vi "呈现图片.vi"(8 "error in (no error)":errorcluster caption="错误输入（无错误）", 11 "直线 输入":refnum<class "直线.lvclass"> caption="DNL_LabVIEW Object in") -> (0 "error out":errorcluster caption="错误输出", 2 "Picture":picture caption="图片", 3 "直线 输出":refnum<class "直线.lvclass"> caption="DNL_LabVIEW Object out")   [LabVIEW 2011, in "直线.lvclass"]
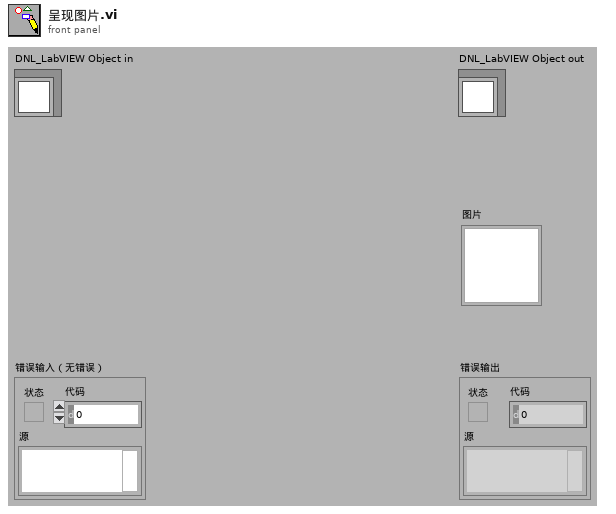
[diagram p1: front panel]
types:
  T1 = typedef "LVPointDoubleTypeDef.ctl" = cluster{"X":dbl, "Y":dbl}
  T2 = cluster{"Width":u16, "Style":enum32{"Solid", "Dash", "Dot", "DashDot", "DashDotDot"}}
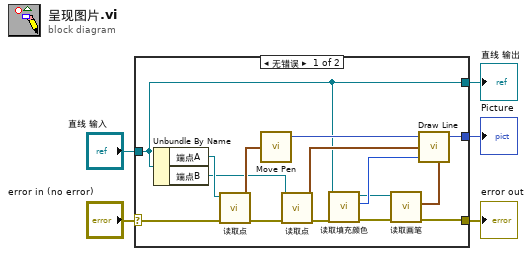
[diagram p0: block diagram]
diagram:
  n1 = case shown="无错误" "error in (no error)" {
    selector: "error in (no error)" -> [w14 w22]
    tunnel: [w7 w22] -> w4
    tunnel: "直线 输入" -> [w11 w21]
    tunnel: [w11 w21] -> w2
    tunnel: [w15 _] -> w1
    frame No Error {
      n2 = Unbundle By Name(w11) -> ("端点A"=w20:refnum<class "点.lvclass">, "端点B"=w18:refnum<class "点.lvclass">)
      n3 = call "读取点.vi"("error in (no error)"=w14, "点输入"=w20) -> ("error out"=w13:errorcluster, "点"=w19:T1)  [unwired: 7 in, 1 out]
      n4 = call <vilib>:"Move Pen.vi"("new position"=w19) -> ("new picture"=w16:picture)  [unwired: 2 in, 2 out]
      n5 = call "读取点.vi"("error in (no error)"=w13, "点输入"=w18) -> ("error out"=w12:errorcluster, "点"=w17:T1)  [unwired: 7 in, 1 out]
      n6 = call "读取填充颜色.vi"("error in (no error)"=w12, "图形输入"=w11) -> ("error out"=w9:errorcluster, "填充颜色"=w10:u32, "图形输出"=w8:refnum<class "直线.lvclass">)  [unwired: 7 in]
      n7 = call "读取画笔.vi"("error in (no error)"=w9, "图形输入"=w8) -> ("error out"=w7:errorcluster, "画笔"=w6:T2)  [unwired: 7 in, 1 out]
      n8 = call <vilib>:"Draw Line.vi"("picture"=w16, "end point"=w17, "color(black)"=w10, "pen"=w6) -> ("new picture"=w15:picture)  [unwired: 1 in, 4 out]
    }
    frame Error {
    }
  }
  "error out" <- w4
  "直线 输出" <- w2
  "Picture" <- w1
